vi "Set Precision(SubVI).vi"(4 "Error In":errorcluster, 6 "Precision":enum16{"Low (Fast)", "Normal", "High (Slow)"}(ring)=enum."Normal", 7 "ModHandle In":T1 {"ModHandle" format="0x%08x"; "Conn" format="0x%08x"}) -> (0 "Error Out":errorcluster, 3 "ModHandle Out":T1 {"ModHandle" format="0x%08x"; "Conn" format="0x%08x"})   [LabVIEW 2019]
doc: "This VI is used to set measurement precision."
uses:
  <instrlib>/Zurich Instruments LabOne/Public/Modules/ziTypeModHandle.ctl
  <instrlib>/Zurich Instruments LabOne/Public/Modules/ziModSetValueDoubleArray.vi
  <instrlib>/Zurich Instruments LabOne/Zurich Instruments LabOne.lvlib
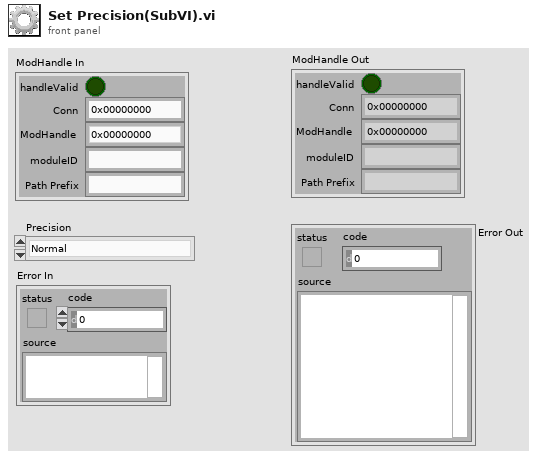
[diagram p1: front panel]
types:
  T1 = typedef "Zurich Instruments LabOne.lvlib/ziTypeModHandle.ctl" = cluster{"handleValid":bool, "Conn":u64, "ModHandle":u64, "moduleID":string, "Path Prefix":string}
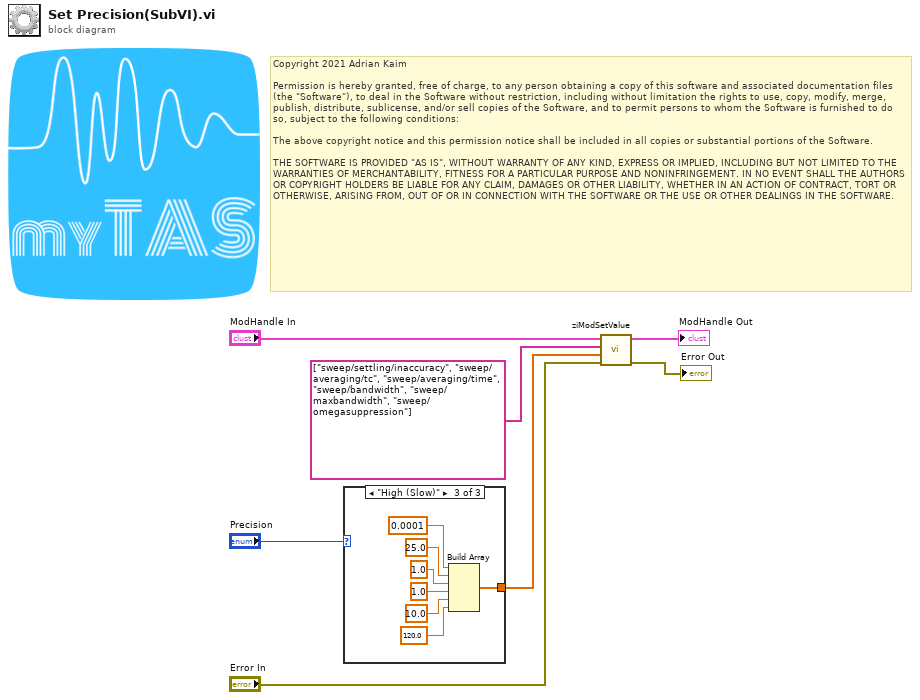
[diagram p0: block diagram]
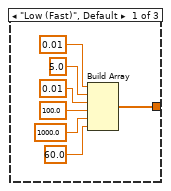
[diagram p2: hidden frame]
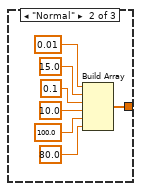
[diagram p3: hidden frame]
diagram:
  # "Copyright 2021 Adrian Kaim\n\nPermission is hereby granted, free of charge, to any person obtaining a copy of this software and associated documentation files (the \"Software\"), to deal in the Software without restriction, including without limitation the rights to use, copy, modify, merge, publish, distribute, sublicense, and/or sell copies of the Software, and to permit persons to whom the Software is furnished to do so, subject to the following conditions:\n\nThe above copyright notice and this permission notice shall be included in all copies or substantial portions of the Software.\n\nTHE SOFTWARE IS PROVIDED \"AS IS\", WITHOUT WARRANTY OF ANY KIND, EXPRESS OR IMPLIED, INCLUDING BUT NOT LIMITED TO THE WARRANTIES OF MERCHANTABILITY, FITNESS FOR A PARTICULAR PURPOSE AND NONINFRINGEMENT. IN NO EVENT SHALL THE AUTHORS OR COPYRIGHT HOLDERS BE LIABLE FOR ANY CLAIM, DAMAGES OR OTHER LIABILITY, WHETHER IN AN ACTION OF CONTRACT, TORT OR OTHERWISE, ARISING FROM, OUT OF OR IN CONNECTION WITH THE SOFTWARE OR THE USE OR OTHER DEALINGS IN THE SOFTWARE."
  n1 = case shown="\"High (Slow)\"" "Precision" {
    tunnel: [w8 w15 w22] -> w5
    frame "Low (Fast)", Default {
      n2 = Build Array(0.01 ("element"), 5.0 ("element"), 0.01 ("element"), 100.0 ("element"), 1000.0 ("element"), 60.0 ("element")) -> (w8:dbl[])
    }
    frame "Normal" {
      n3 = Build Array(0.01 ("element"), 15.0 ("element"), 0.1 ("element"), 10.0 ("element"), 100.0 ("element"), 80.0 ("element")) -> (w15:dbl[])
    }
    frame "High (Slow)" {
      n4 = Build Array(0.0001 ("element"), 25.0 ("element"), 1.0 ("element"), 1.0 ("element"), 10.0 ("element"), 120.0 ("element")) -> (w22:dbl[])
    }
  }
  n5 = call-poly <instrlib>:"ziModSetValue.vi"("Error In"="Error In", "Values"=w5, "Paths"=string[] ["sweep/settling/inaccuracy", "sweep/averaging/tc", "sweep/averaging/time", "sweep/bandwidth", "sweep/maxbandwidth", "sweep/omegasuppression"], "ModHandle In"="ModHandle In") -> ("Error Out"=→"Error Out":errorcluster, "ModHandle Out"=→"ModHandle Out":T1)  [unwired: 6 in]
